vi "Find Port.vi"(8 "error in":errorcluster, 10 "port":u32, 11 "Ballard ARINC 429 ref":T1 format="%.0x") -> (0 "error out":errorcluster, 2 "port ref":T1 format="%.0x", 3 "Ballard ARINC 429 ref out":T1 format="%.0x", 4 "found?":bool)   [LabVIEW 2020, in "Ballard ARINC 429 Scripting.lvlib"]
uses:
  Ballard ARINC 429 Scripting.lvlib
  ARINC 429/ARINC 429 Scripting.lvlib
  <vilib>/NI VeriStand/Custom Device API/Custom Device Item Ref.ctl
  <vilib>/NI VeriStand/Custom Device API/Custom Device API.lvlib
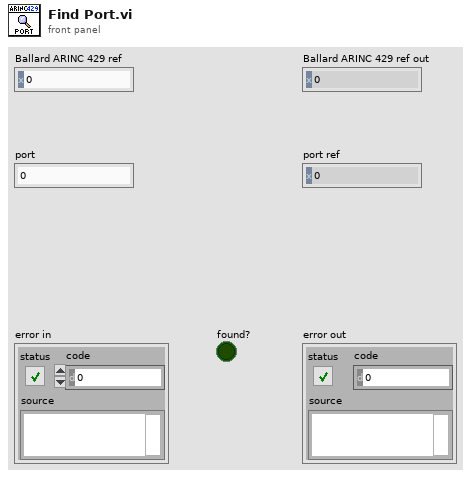
[diagram p1: front panel]
types:
  T1 = typedef "Custom Device API.lvlib/Custom Device Item Ref.ctl" = u64
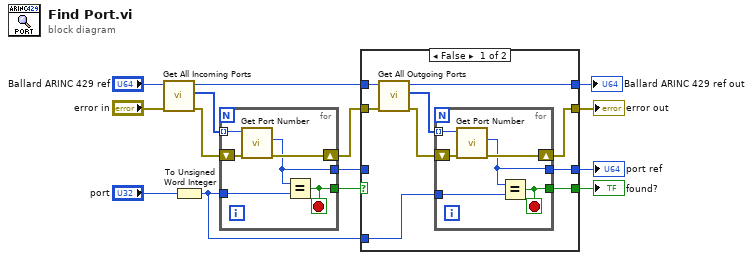
[diagram p0: block diagram]
diagram:
  n1 = call "Get All Incoming Ports.vi"("error in"="error in", "Ballard ARINC 429 ref"="Ballard ARINC 429 ref") -> ("error out"=w8:errorcluster, "Port refs"=w9:T1[], "Ballard ARINC 429 ref out"=w13:T1)  [unwired: 7 in]
  n2 = To Unsigned Word Integer(number="port") -> (unsigned 16bit integer=w1:u16)
  n3 = for {
    tunnel: w9 -> [w20] mode=indexing
    shift-right: [w18] -> w5
    shift-left: w8 -> [w19]
    tunnel: w1 -> [w17]
    tunnel: [w16] -> w6
    tunnel: [w15] -> w4
    stop <- w16 stop-if-true
    n4 = call "Get Port Number.vi"("error in"=w19, "port ref in"=w20) -> ("error out"=w18:errorcluster, "port number"=w15:u16)  [unwired: 6 in, 2 out]
    n5 = Equal?(x=w15, y=w17) -> (x = y?=w16:bool)
  }
  n6 = case shown="False" w6 {
    selector: w6 -> [_ w36]
    tunnel: w13 -> [w29 w39]
    tunnel: [w28 w39] -> w12
    tunnel: [w21 w38] -> w10
    tunnel: w5 -> [w27 w38]
    tunnel: w4 -> [_ w37]
    tunnel: [w26 w37] -> w3
    tunnel: [w22 w36] -> w2
    tunnel: w1 -> [w23 _]
    frame False {
      n7 = call "Get All Outgoing Ports.vi"("error in"=w27, "Ballard ARINC 429 ref"=w29) -> ("error out"=w25:errorcluster, "Port refs"=w24:T1[], "Ballard ARINC 429 ref out"=w28:T1)  [unwired: 7 in]
      n8 = for {
        tunnel: w24 -> [w35] mode=indexing
        shift-right: [w33] -> w21
        shift-left: w25 -> [w34]
        tunnel: w23 -> [w32]
        tunnel: [w31] -> w22
        tunnel: [w30] -> w26
        stop <- w31 stop-if-true
        n9 = call "Get Port Number.vi"("error in"=w34, "port ref in"=w35) -> ("error out"=w33:errorcluster, "port number"=w30:u16)  [unwired: 6 in, 2 out]
        n10 = Equal?(x=w30, y=w32) -> (x = y?=w31:bool)
      }
    }
    frame True {
    }
  }
  "port ref" <- w3
  "error out" <- w10
  "Ballard ARINC 429 ref out" <- w12
  "found?" <- w2
